vi "BioMapT2mWriter.vi"(5 "TrigDelay":dbl, 7 "time bin (s)":dbl=0.001, 8 "error in":errorcluster, 9 "SpecDepth":u16, 10 "mzArray":dbl[](array[numeric])=[0.0, 1.0, 0.0], 11 "image file path":path) -> (0 "error out":errorcluster)   [LabVIEW 2013]
panel:
  out "result":dbl[](array[numeric])
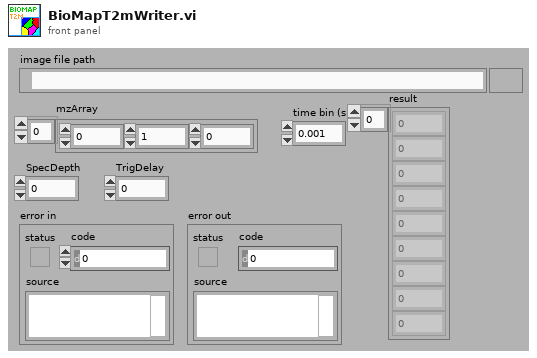
[diagram p1: front panel]
types:
  T1 = enum16{"big-endian, network order", "native, host order", "little-endian"}
  T2 = enum16{"open", "replace", "create", "open or create", "replace or create", "replace or create with confirmation"}
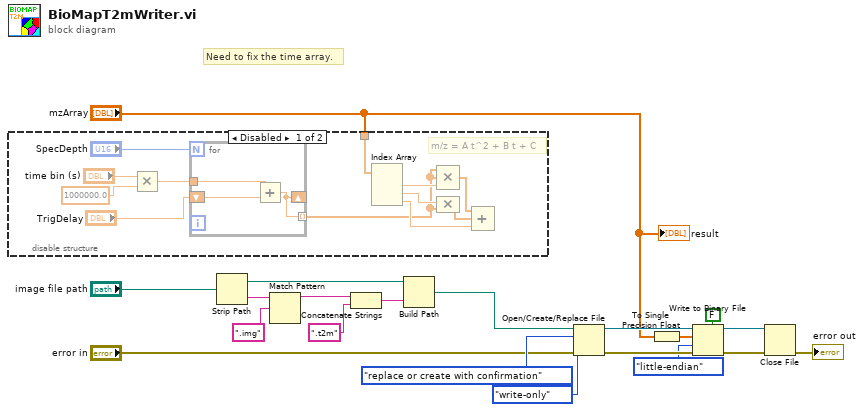
[diagram p0: block diagram]
diagram:
  # "Need to fix the time array."
  n1 = disable-structure shown="Disabled" {
    disable-tunnel: "mzArray" -> [w21 _]
    frame Disabled {
      # "m/z = A t^2 + B t + C"
      n2 = Multiply(x="time bin (s)", y=1000000.0) -> (x*y=w22:dbl)
      n3 = for {
        N: "SpecDepth" -> [_]
        shift-right: [w34] -> _
        shift-left: "TrigDelay" -> [w35]
        tunnel: [w34] -> w26 mode=indexing
        tunnel: w22 -> [w33]
        n4 = Add(x=w33, y=w35) -> (x+y=w34:dbl)
      }
      n5 = Index Array(array=w21) -> (element #1=w27:dbl, element #2=w28:dbl, element #3=w29:dbl)  [unwired: 3 in]
      n6 = Compound Arithmetic op=MULTIPLY(w26, w26, w27) -> (w31:dbl[])
      n7 = Compound Arithmetic op=MULTIPLY(w28, w26) -> (w30:dbl[])
      n8 = Compound Arithmetic op=ADD(w31, w30, w29) -> ()  [unwired: 1 out]
    }
    frame Enabled {
    }
  }
  n9 = Strip Path(path="image file path") -> (stripped path=w6:path, name=w10:string)
  n10 = Match Pattern(string=w10, regular expression=".img" ("string")) -> (before substring=w9:string)  [unwired: 1 in, 3 out]
  n11 = Concatenate Strings(w9, ".t2m" ("string")) -> (w7:string)
  n12 = Build Path(base path=w6, name or relative path=w7) -> (appended path=w5:path)
  n13 = Open/Create/Replace File(file path (use dialog)=w5, error in="error in", operation (0:open)=T2."replace or create with confirmation", access (0:read/write)=enum16{"read/write", "read-only", "write-only"}."write-only") -> (refnum out=w18:refnum<file>, error out=w15:errorcluster)  [unwired: 2 in, 1 out]
  n14 = To Single Precision Float(number="mzArray") -> (single precision float=w20:sgl[])
  n15 = Write to Binary File(file (use dialog)=w18, data=w20, error in=w15, 5:FALSE ("prepend array or string size? (T)"), 9:T1."little-endian" ("byte order (0:big-endian, network order)")) -> (refnum out=w13:refnum<file>, error out=w14:errorcluster)  [unwired: 1 in, 1 out]
  n16 = Close File(refnum=w13, error in=w14) -> (error out=→"error out":errorcluster)  [unwired: 1 out]
  "result" <- "mzArray"
